vi "Main.vi"(11 "Module Admin":refnum<class "Delacor_lib_QMH_Module Admin.lvclass">) -> ()   [LabVIEW 2024, in "Singleton Subpanel.lvlib"]
doc: "This template is based off of the Queued Message Handler design pattern and the Queued Message Handler project template that ships with LabVIEW.\n\nThe main difference is that the queue is private to this module and communication between modules is performed via Broadcast and Request events.\n\nRequest events are wrapped in public API methods and are handled in the Event Handling Loop (EHL) of this VI. Any module can register for Broadcast events sent by this module. The EHL generates messages based on user interface actions.\n\nThe Message Handling Loop (MHL) processes messages generated by the EHL, or by other messages. The messages are string values, so new messages can be added easily to the Message Cases case structure in the MHL. Each message cluster can also provide an optional value for Message Data, which is a variant that can be converted to whatever message-specific data is required.\n_____\nBased on DQMH Dev Tools: Project Template 7.1.0.1499."
uses:
  Singleton Subpanel.lvlib
  <vilib>/Delacor/Delacor QMH/Libraries/Module Admin_class/Delacor_lib_QMH_Module Admin.lvclass
  Module Data--cluster.ctl
  <vilib>/Delacor/Delacor QMH/Libraries/Message Queue_class/Delacor_lib_QMH_Message Queue.lvclass/Delacor_lib_QMH_Message Queue.ctl
  Stop Argument--cluster.ctl
  <vilib>/Delacor/Delacor QMH/Libraries/Module Admin_class/Delacor_lib_QMH_Module Admin.lvclass/Delacor_lib_QMH_Module Admin.ctl
  Draw FP in SubPanel Argument--cluster.ctl
  Remove from SubPanel Argument--cluster.ctl
  <vilib>/Utility/miscctls.llb/LVPointTypeDef.ctl
  <vilib>/Delacor/Delacor QMH/Libraries/Message Queue_class/Delacor_lib_QMH_Enqueue Message (Single).vi
  <vilib>/Delacor/Delacor QMH/Libraries/Module Admin_class/Delacor_lib_QMH_Get External Launch.vi
  <vilib>/Delacor/Delacor QMH/Libraries/Message Queue_class/Delacor_lib_QMH_Message Queue.lvclass
panel:
  out "error out":errorcluster
  out "Status":string
  in  "Simulate MHL Error":bool
  in  "Simulate EHL Error":bool
  # "Other processes communicate with this Module via its Public API (wrappers for its Request Events).\n\nThis Module communicates with other processes via its Broadcast Events.\nAny process that wants to receive these messages can register for this module's Broadcast events."
  # "This template is for the DQMH framework. See the block diagram for more information on how to use this template."
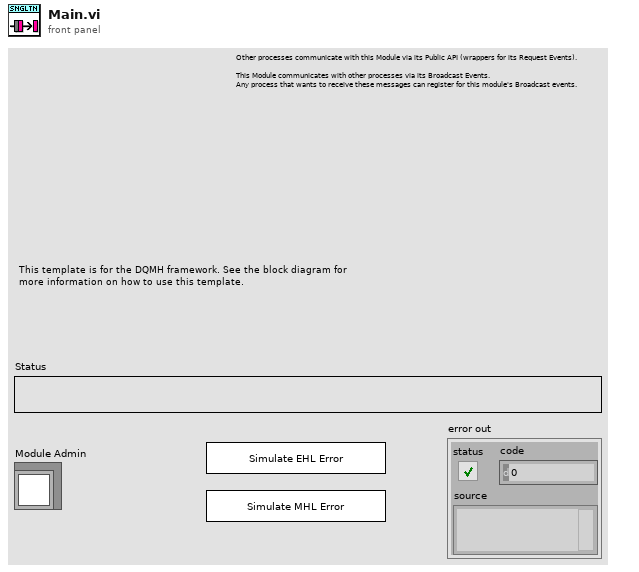
[diagram p1: front panel]
types:
  T1 = typedef "Singleton Subpanel.lvlib/Request Events--cluster.ctl" = cluster{"Stop Module":refnum<user-event>, "Show Panel":refnum<user-event>, "Hide Panel":refnum<user-event>, "Get Module Execution Status":refnum<user-event>, "Show Diagram":refnum<user-event>, "Draw FP in SubPanel":refnum<user-event>, "Remove from SubPanel":refnum<user-event>}
  T2 = typedef "Singleton Subpanel.lvlib/Module Data--cluster.ctl" = cluster{"Status":string, "Sub Panel":refnum<vi>}
  T3 = enum32{"invalid lock state", "Not Locked", "Locked (No Password)", "Password-protected"}
  T4 = typedef "Singleton Subpanel.lvlib/Stop Argument--cluster.ctl" = cluster{"Origin":string, "Exit via Stop Module Req?":bool, "Wait for Module to stop?":bool}
  T5 = typedef "Singleton Subpanel.lvlib/Draw FP in SubPanel Argument--cluster.ctl" = cluster{"Sub Panel":refnum<vi>}
  T6 = typedef "Singleton Subpanel.lvlib/Remove from SubPanel Argument--cluster.ctl" = cluster{"Boolean":bool}
  T7 = typedef "LVPointTypeDef.ctl" = cluster{"Horizontal":i16, "Vertical":i16}
  T8 = enum32{"Invalid", "Standard", "Closed", "Hidden", "Minimized", "Maximized"}
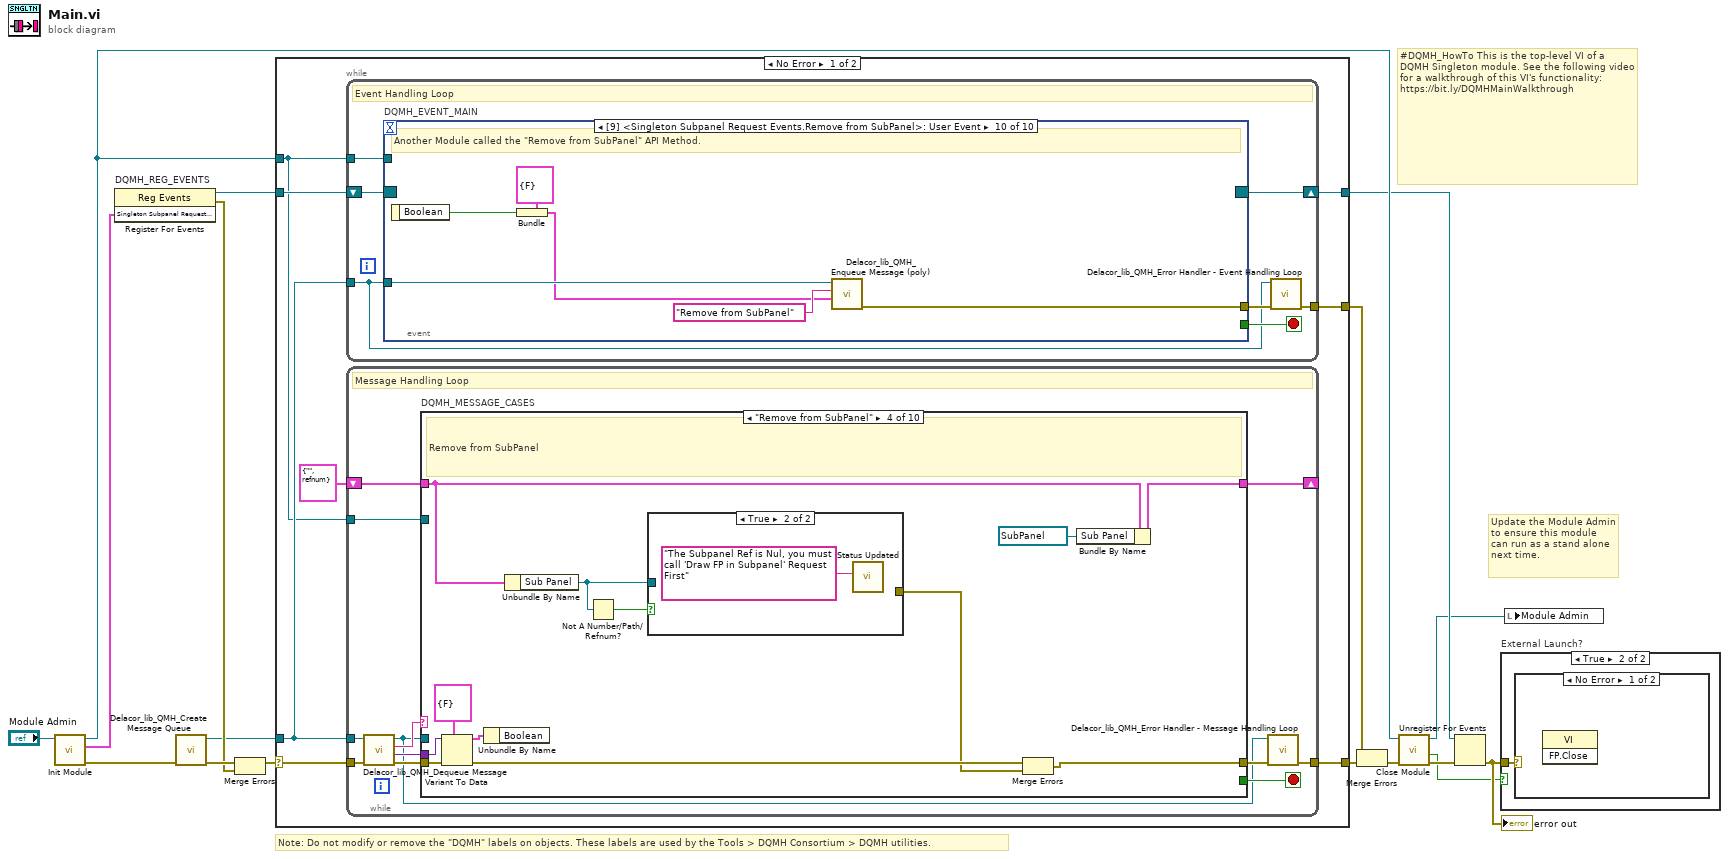
[diagram p0: block diagram]
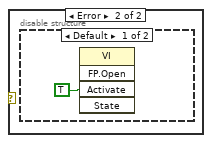
[diagram p3: hidden frame]
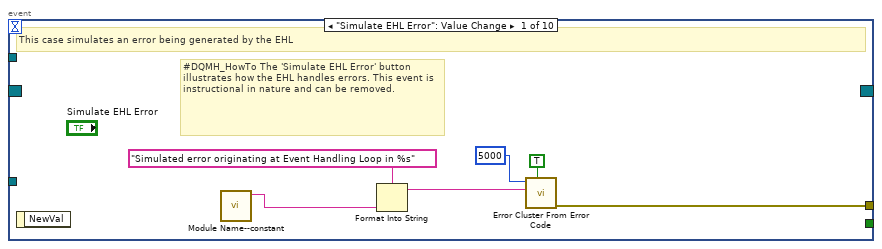
[diagram p5: hidden frame]
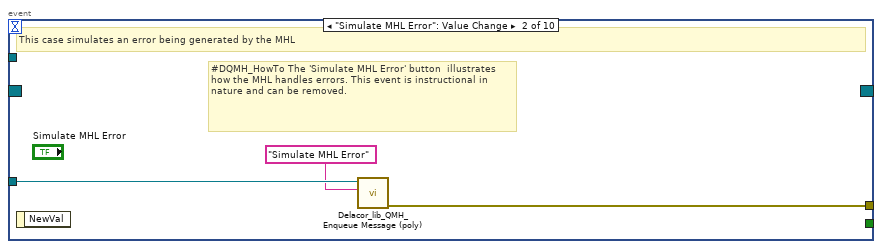
[diagram p6: hidden frame]
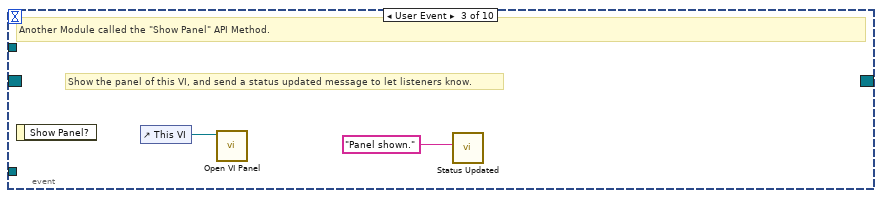
[diagram p7: hidden frame]
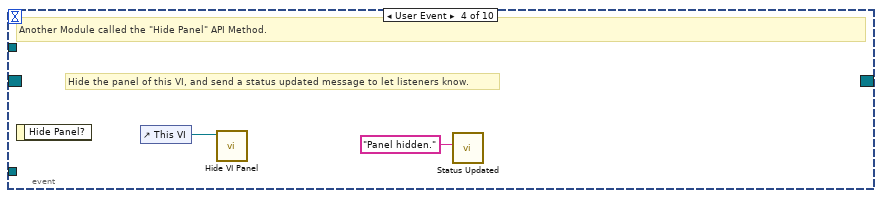
[diagram p8: hidden frame]
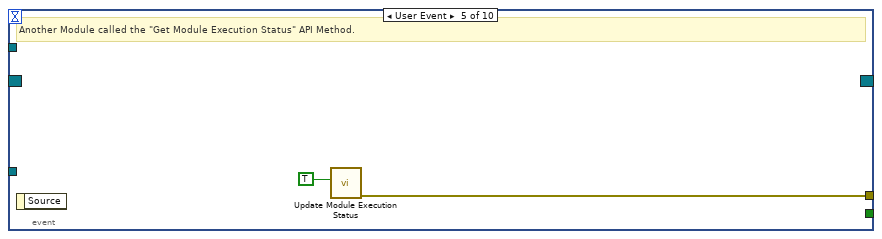
[diagram p9: hidden frame]
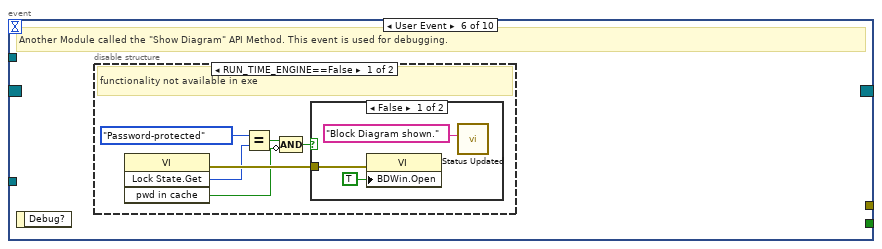
[diagram p10: hidden frame]
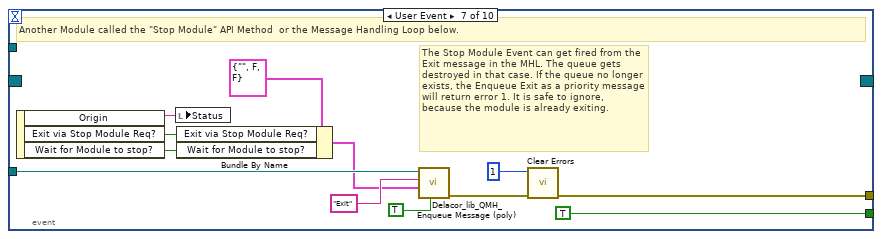
[diagram p13: hidden frame]
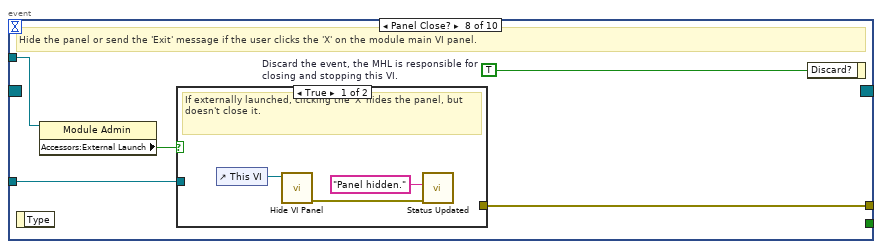
[diagram p14: hidden frame]
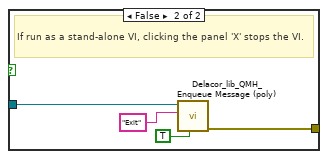
[diagram p15: hidden frame]
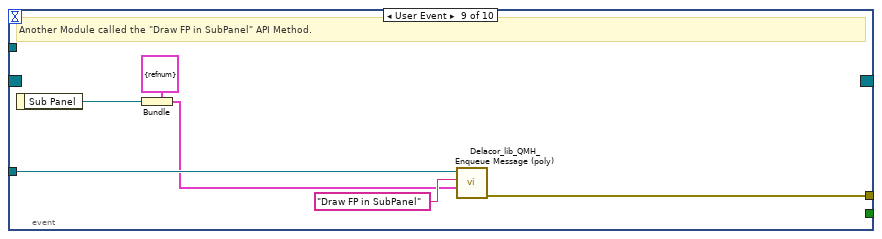
[diagram p16: hidden frame]
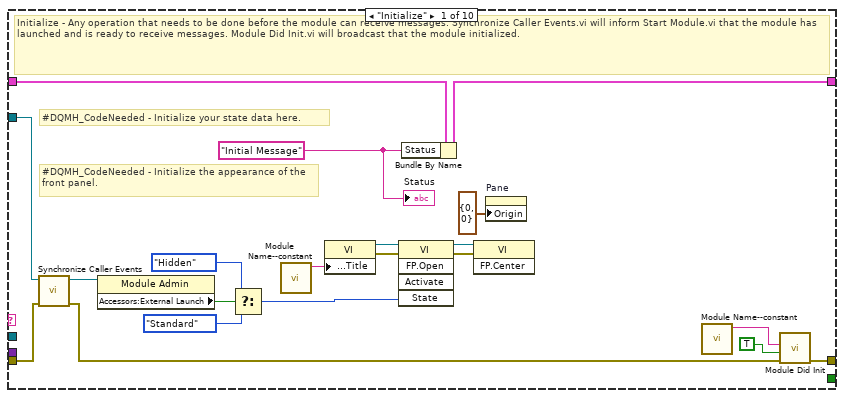
[diagram p17: hidden frame]
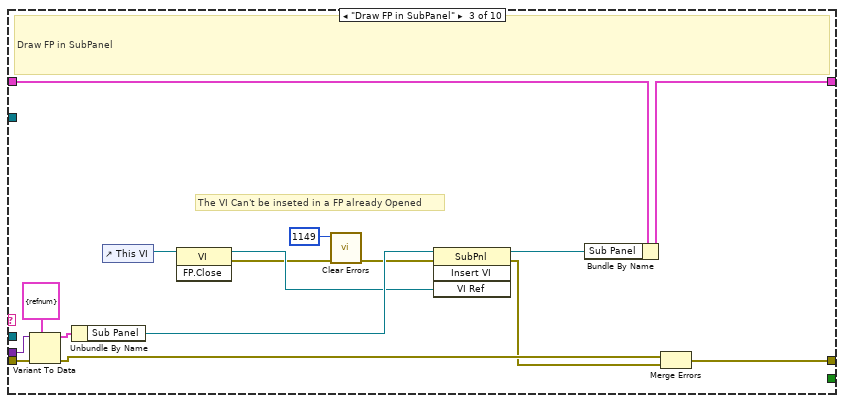
[diagram p19: hidden frame]
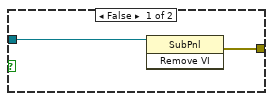
[diagram p20: hidden frame]
diagram:
  # "#DQMH_HowTo This is the top-level VI of a DQMH Singleton module. See the following video for a walkthrough of this VI's functionality: https://bit.ly/DQMHMainWalkthrough"
  # "Note: Do not modify or remove the \"DQMH\" labels on objects. These labels are used by the Tools > DQMH Consortium > DQMH utilities."
  # "Update the Module Admin to ensure this module can run as a stand alone next time."
  n1 = call "Init Module.vi"("Singleton Module Admin in"="Module Admin") -> ("error out"=w16:errorcluster, "Singleton Subpanel Request Events"=w5:T1, "Singleton Module Admin out"=w8:refnum<class "Delacor_lib_QMH_Module Admin.lvclass">)  [unwired: 8 in]
  n2 = register-events "DQMH_REG_EVENTS"(w5) -> (reference out=w6:refnum<event-registration>, error out=w9:errorcluster)  [unwired: 2 in]
  n3 = call <vilib>:"Delacor_lib_QMH_Create Message Queue.vi"("error in"=w16) -> ("error out"=w11:errorcluster, "Message Queue"=w4:refnum<class "Delacor_lib_QMH_Message Queue.lvclass">)  [unwired: 9 in]
  n4 = Merge Errors(w11, w9) -> (w10:errorcluster)
  n5 = case shown="No Error" w10 {
    selector: w10 -> [w23 w222]
    tunnel: [w25 w221] -> w17
    tunnel: [w22 w220] -> w7
    tunnel: w6 -> [w20 w220]
    tunnel: w4 -> [w19 w215]
    tunnel: [w24 _] -> w14
    tunnel: w8 -> [w18 w216]
    frame No Error {
      n6 = while {
        tunnel: w19 -> [w26]
        shift-right: [w29] -> w22
        shift-left: w20 -> [w30]
        tunnel: [w31] -> w24
        tunnel: w18 -> [w27]
        stop <- w28 stop-if-true
        # "Event Handling Loop"
        n7 = event "DQMH_EVENT_MAIN" shown="[9] <Singleton Subpanel Request Events.Remove from SubPanel>: User Event" {
          selector: w30 -> [_ _ _ _ _ _ _ _ _ _]
          dyn-events: [_ _ _ _ _ _ _ _ _ _] -> w29
          timeout: _ -> [_ _ _ _ _ _ _ _ _ _]
          tunnel: [_ _ _ _ _ _ TRUE ("Discard?") _ _ _] -> w28
          tunnel: w26 -> [_ w40 _ _ _ _ w64 w71 w86 w92]
          tunnel: [w38 w41 _ _ w47 _ w67 w73 w81 w87] -> w32
          tunnel: w27 -> [_ _ _ _ _ _ _ w70 _ _]
          event "Simulate EHL Error": Value Change {
            # "#DQMH_HowTo The 'Simulate EHL Error' button  illustrates how the EHL handles errors. This event is instructional in nature and can be removed."
            # "This case simulates an error being generated by the EHL"
            n8 = event-data() -> ()  [unwired: 1 in, 1 out]
            n9 = call "Module Name--constant.vi"() -> ("Module Name"=w35:string)  [unwired: 11 in]
            n10 = Format Into String(format string="Simulated error originating at Event Handling Loop in %s", w35) -> (resulting string=w36:string)  [unwired: 2 in, 1 out]
            n11 = call <vilib>:"Error Cluster From Error Code.vi"("show call chain? (False)"=TRUE, "error message (\"\")"=w36, "error code (0)"=5000) -> ("error out"=w38:errorcluster)  [unwired: 6 in]
          }
          event "Simulate MHL Error": Value Change {
            # "#DQMH_HowTo The 'Simulate MHL Error' button  illustrates how the MHL handles errors. This event is instructional in nature and can be removed."
            # "This case simulates an error being generated by the MHL"
            n12 = event-data() -> ()  [unwired: 1 in, 1 out]
            n13 = call-poly <vilib>:"Delacor_lib_QMH_Enqueue Message (poly).vi"("Message"="Simulate MHL Error", "Message Queue in"=w40) -> ("error out"=w41:errorcluster)  [unwired: 8 in, 1 out]
          }
          event User Event {
            # "Show the panel of this VI, and send a status updated message to let listeners know."
            # "Another Module called the \"Show Panel\" API Method."
            n14 = event-data() -> ()  [unwired: 1 in, 1 out]
            n15 = control-ref of="This VI"() -> (w43:refnum<vi>)
            n16 = call "Open VI Panel.vi"("VI"=w43) -> ()  [unwired: 10 in, 1 out]
            n17 = call "Status Updated.vi"("Status"="Panel shown." ("format string")) -> ()  [unwired: 10 in, 1 out]
          }
          event User Event {
            # "Hide the panel of this VI, and send a status updated message to let listeners know."
            # "Another Module called the \"Hide Panel\" API Method."
            n18 = event-data() -> ()  [unwired: 1 in, 1 out]
            n19 = control-ref of="This VI"() -> (w45:refnum<vi>)
            n20 = call "Hide VI Panel.vi"("VI"=w45) -> ()  [unwired: 10 in, 1 out]
            n21 = call "Status Updated.vi"("Status"="Panel hidden." ("format string")) -> ()  [unwired: 10 in, 1 out]
          }
          event User Event {
            # "Another Module called the \"Get Module Execution Status\" API Method."
            n22 = event-data() -> ()  [unwired: 1 in, 1 out]
            n23 = call "Update Module Execution Status.vi"("Running?"=TRUE) -> ("error out"=w47:errorcluster)  [unwired: 10 in]
          }
          event User Event {
            # "Another Module called the \"Show Diagram\" API Method. This event is used for debugging."
            n24 = event-data() -> ()  [unwired: 1 in, 1 out]
            n25 = disable-structure shown="RUN_TIME_ENGINE==False" {
              frame condition #0 (active) {
                # "functionality not available in exe"
                n26 = invoke on="Invoke Node" class="VI" method="Lock State.Get"() -> (error out=w53:errorcluster, "Get Lock State"=w52:T3, "pwd in cache"=w49:bool)  [unwired: 4 in, 1 out]
                n27 = Equal?(x=T3."Password-protected", y=w52) -> (x = y?=w50:bool)
                n28 = Compound Arithmetic op=AND(w50, invert w49) -> (w48:bool)
                n29 = case shown="False" w48 {
                  tunnel: w53 -> [w56 _]
                  frame False {
                    n30 = property on="Property Node" class="VI"(error in=w56, "BDWin.Open"=TRUE ("Block Diagram Window:Open")) -> ()  [unwired: 1 in, 2 out]
                    n31 = call "Status Updated.vi"("Status"="Block Diagram shown." ("format string")) -> ()  [unwired: 10 in, 1 out]
                  }
                  frame True {
                    # "Password-protected VI, and the password is not in the cache. Do not show the diagram."
                  }
                }
              }
              frame condition #1 {
              }
            }
          }
          event User Event {
            # "The Stop Module Event can get fired from the Exit message in the MHL. The queue gets destroyed in that case. If the queue no longer exists, the Enqueue Exit as a priority message will return error 1. It is safe to ignore, because the module is already exiting."
            # "Another Module called the \"Stop Module\" API Method  or the Message Handling Loop below."
            n32 = event-data() -> ("Origin"=w63:string, "Exit via Stop Module Req?"=w59:bool, "Wait for Module to stop?"=w58:bool)  [unwired: 1 in]
            n33 = local write "Status"(w63) -> ()
            n34 = Bundle By Name(cluster=T4 {"Origin"="", "Exit via Stop Module Req?"=FALSE, "Wait for Module to stop?"=FALSE} ("Stop Argument"), "Exit via Stop Module Req?"=w59, "Wait for Module to stop?"=w58) -> (w57:T4)
            n35 = call-poly <vilib>:"Delacor_lib_QMH_Enqueue Message (poly).vi"("Priority Message? (F)"=TRUE, "Message Data"=w57, "Message"="Exit", "Message Queue in"=w64) -> ("error out"=w68:errorcluster)  [unwired: 6 in, 1 out]
            n36 = call <vilib>:"Clear Errors.vi"("error in (no error)"=w68, "specific error code to clear (0: all)"=1) -> ("error out"=w67:errorcluster)  [unwired: 4 in, 1 out]
          }
          event Panel Close? {
            w72 = TRUE  # Discard the event, the MHL is responsible for closing and stopping this VI.
            # "Hide the panel or send the 'Exit' message if the user clicks the 'X' on the module main VI panel."
            n37 = event-data() -> ()  [unwired: 1 in, 1 out]
            n38 = property on="Property Node" class="Module Admin"(reference=w70) -> ("Accessors:External Launch"=w69:bool)  [unwired: 1 in, 2 out]
            n39 = case shown="True" w69 {
              tunnel: w71 -> [_ w79]
              tunnel: [_ w80] -> w73
              frame True {
                # "If externally launched, clicking the 'X' hides the panel, but doesn't close it."
                n40 = control-ref of="This VI"() -> (w76:refnum<vi>)
                n41 = call "Hide VI Panel.vi"("VI"=w76) -> ("error out"=w74:errorcluster)  [unwired: 10 in]
                n42 = call "Status Updated.vi"("error in"=w74, "Status"="Panel hidden." ("format string")) -> ()  [unwired: 9 in, 1 out]
              }
              frame False {
                # "If run as a stand-alone VI, clicking the panel 'X' stops the VI."
                n43 = call-poly <vilib>:"Delacor_lib_QMH_Enqueue Message (poly).vi"("Priority Message? (F)"=TRUE, "Message"="Exit", "Message Queue in"=w79) -> ("error out"=w80:errorcluster)  [unwired: 7 in, 1 out]
              }
            }
            n44 = event-data ("Event Filter Node")("Discard?"=w72) -> ()  [unwired: 1 in, 1 out]
          }
          event User Event {
            # "Another Module called the \"Draw FP in SubPanel\" API Method."
            n45 = event-data() -> ("Sub Panel"=w82:refnum<vi>)  [unwired: 1 in]
            n46 = Bundle(cluster=T5 {"Sub Panel"=refnum} ("Draw FP in SubPanel Argument"), "Sub Panel"=w82) -> (w83:T5)
            n47 = call-poly <vilib>:"Delacor_lib_QMH_Enqueue Message (poly).vi"("Message Data"=w83, "Message"="Draw FP in SubPanel", "Message Queue in"=w86) -> ("error out"=w81:errorcluster)  [unwired: 7 in, 1 out]
          }
          event User Event {
            # "Another Module called the \"Remove from SubPanel\" API Method."
            n48 = event-data() -> ("Boolean"=w88:bool)  [unwired: 1 in]
            n49 = Bundle(cluster=T6 {"Boolean"=FALSE} ("Remove from SubPanel Argument"), "Boolean"=w88) -> (w89:T6)
            n50 = call-poly <vilib>:"Delacor_lib_QMH_Enqueue Message (poly).vi"("Message Data"=w89, "Message"="Remove from SubPanel", "Message Queue in"=w92) -> ("error out"=w87:errorcluster)  [unwired: 7 in, 1 out]
          }
        }
        n51 = call-dynamic "Delacor_lib_QMH_Error Handler - Event Handling Loop.vi"("error in"=w32, "Message Queue in"=w26) -> ("dup error in"=w31:errorcluster)  [unwired: 8 in, 1 out]
      }
      n52 = while {
        tunnel: w19 -> [w93]
        shift-right: [w101] -> _
        shift-left: T2 {"Status"="", "Sub Panel"=refnum} ("Data Cluster") -> [w102]
        tunnel: w23 -> [w104]
        tunnel: [w96] -> w25
        tunnel: w18 -> [w97]
        stop <- w100 stop-if-true
        # "Message Handling Loop"
        n53 = call-dynamic "Delacor_lib_QMH_Dequeue Message.vi"("error in"=w104, "Message Queue in"=w93) -> ("error out"=w103:errorcluster, "Message Data"=w98:variant, "Message"=w99:string, "Message Queue out"=w94:refnum<class "Delacor_lib_QMH_Message Queue.lvclass">)  [unwired: 6 in]
        n54 = case "DQMH_MESSAGE_CASES" shown="\"Remove from SubPanel\"" w99 {
          selector: w99 -> [_ _ _ _ _ _ _ _ _ w210]
          tunnel: w94 -> [_ _ _ _ _ _ _ w175 w198 _]
          tunnel: w103 -> [w122 w126 w142 w154 w160 w162 w171 w182 w204 w213]
          tunnel: [w120 w126 w132 w148 w159 w162 w170 w178 w199 w214] -> w95
          tunnel: w102 -> [w111 w125 w141 w149 w158 w161 w168 w177 w190 w211]
          tunnel: [w110 w125 w128 w144 w158 w161 w168 w177 w190 w211] -> w101
          tunnel: [_ _ _ _ _ _ _ _ w197 _] -> w100
          tunnel: w98 -> [_ _ w140 w152 _ _ _ w176 w196 _]
          tunnel: w97 -> [w112 _ _ _ _ _ _ w174 w191 _]
          frame "Initialize" {
            w106 = "Initial Message" ("Initial Message")
            # "#DQMH_CodeNeeded - Initialize the appearance of the front panel."
            # "#DQMH_CodeNeeded - Initialize your state data here."
            # "Initialize - Any operation that needs to be done before the module can receive messages. Synchronize Caller Events.vi will inform Start Module.vi that the module has launched and is ready to receive messages. Module Did Init.vi will broadcast that the module initialized."
            n55 = call "Synchronize Caller Events.vi"("error in"=w122, "Singleton Module Admin in"=w112) -> ("error out"=w121:errorcluster, "Singleton Module Admin out"=w107:refnum<class "Delacor_lib_QMH_Module Admin.lvclass">)  [unwired: 8 in]
            n56 = property on="Property Node" class="Module Admin"(reference=w107) -> ("Accessors:External Launch"=w116:bool)  [unwired: 1 in, 2 out]
            n57 = Select(t=T8."Hidden" ("State"), s=w116, f=T8."Standard" ("State")) -> (s? t:f=w113:T8)
            n58 = call "Module Name--constant.vi"() -> ("Module Name"=w119:string)  [unwired: 11 in]
            n59 = property on="Property Node" class="VI"("Front Panel.Title"=w119) -> (reference out=w118:refnum<vi>, error out=w124:errorcluster)  [unwired: 2 in]
            n60 = invoke on="Invoke Node" class="VI" method="FP.Open"(reference=w118, error in=w124, "State"=w113) -> (reference out=w117:refnum<vi>, error out=w123:errorcluster)  [unwired: 2 in, 3 out]
            n61 = Bundle By Name(cluster=w111, "Status"=w106) -> (w110:T2)
            n62 = invoke on="Invoke Node" class="VI" method="FP.Center"(reference=w117, error in=w123) -> ()  [unwired: 1 in, 3 out]
            n63 = property on="Pane" class="Pane"("Origin"=T7 {"Horizontal"=0, "Vertical"=0}) -> ()  [unwired: 2 in, 2 out]
            n64 = call "Module Name--constant.vi"() -> ("Module Name"=w108:string)  [unwired: 11 in]
            n65 = call "Module Did Init.vi"("error in"=w121, "Initialized?"=TRUE, "Origin"=w108) -> ("error out"=w120:errorcluster)  [unwired: 8 in]
            "Status" <- w106
          }
          frame "---Module Specific---" {
            # "Separator -- The following cases handle messages specific to this Module."
          }
          frame "Draw FP in SubPanel" {
            # "The VI Can't be inseted in a FP already Opened"
            # "Draw FP in SubPanel"
            n66 = Variant To Data(error in=w142, type=T5 {"Sub Panel"=refnum} ("Draw FP in SubPanel Argument"), Variant=w140) -> (data=w138:T5, error out=w131:errorcluster)
            n67 = Unbundle By Name(w138) -> ("Sub Panel"=w136:refnum<vi>)
            n68 = control-ref of="This VI"() -> (w137:refnum<vi>)
            n69 = invoke class="VI" method="FP.Close"(reference=w137) -> (reference out=w135:refnum<vi>, error out=w134:errorcluster)  [unwired: 2 in, 1 out]
            n70 = call <vilib>:"Clear Errors.vi"("error in (no error)"=w134, "specific error code to clear (0: all)"=1149) -> ("error out"=w133:errorcluster)  [unwired: 4 in, 1 out]
            n71 = invoke class="SubPnl" method="Insert VI"(reference=w136, error in=w133, "VI Ref"=w135) -> (reference out=w127:refnum<vi>, error out=w130:errorcluster)  [unwired: 1 in, 2 out]
            n72 = Bundle By Name(cluster=w141, "Sub Panel"=w127) -> (w128:T2)
            n73 = Merge Errors(w131, w130) -> (w132:errorcluster)
          }
          frame "Remove from SubPanel" {
            # "Remove from SubPanel"
            n74 = Variant To Data(error in=w154, type=T6 {"Boolean"=FALSE} ("Remove from SubPanel Argument"), Variant=w152) -> (data=w150:T6, error out=w153:errorcluster)
            n75 = Unbundle By Name(w150) -> ()  [unwired: 1 out]
            n76 = Unbundle By Name(w149) -> ("Sub Panel"=w146:refnum<vi>)
            n77 = Not A Number/Path/Refnum?(number/path/refnum=w146) -> (NaN/Path/Refnum?=w145:bool)
            n78 = case shown="True" w145 {
              tunnel: w146 -> [w156 _]
              tunnel: [w155 _] -> w147
              frame False {
                n79 = invoke class="SubPnl" method="Remove VI"(reference=w156) -> (error out=w155:errorcluster)  [unwired: 2 in, 2 out]
              }
              frame True {
                n80 = call "Status Updated.vi"("Status"="The Subpanel Ref is Nul, you must call 'Draw FP in Subpanel' Request First") -> ()  [unwired: 10 in, 1 out]
              }
            }
            n81 = Merge Errors(w153, w147) -> (w148:errorcluster)
            n82 = Bundle By Name(cluster=w149, "Sub Panel"=refnum<vi> refnum) -> (w144:T2)
          }
          frame "---Copy This Frame---" {
            # "Duplicate this frame when creating new messages.  Change this comment in the duplicated frame to describe this message."
            n83 = Merge Errors(w160) -> (w159:errorcluster)
          }
          frame "---Exit and Error Handling---" {
            # "Separator - The following cases handle errors and exit messages."
          }
          frame "Simulate MHL Error" {
            # "#DQMH_HowTo The 'Simulate MHL Error' button  illustrates how the MHL handles errors. This event is instructional in nature and can be removed."
            # "Simulate an error occurring at the MHL"
            n84 = call "Module Name--constant.vi"() -> ("Module Name"=w164:string)  [unwired: 11 in]
            n85 = Format Into String(format string="Simulated error originating at Message Handling Loop in %s", w164) -> (resulting string=w165:string)  [unwired: 2 in, 1 out]
            n86 = call <vilib>:"Error Cluster From Error Code.vi"("show call chain? (False)"=TRUE, "error message (\"\")"=w165, "error code (0)"=5001) -> ("error out"=w169:errorcluster)  [unwired: 6 in]
            n87 = Merge Errors(w171, w169) -> (w170:errorcluster)
          }
          frame "Error" {
            # "#DQMH_CodeRecommended - If the module is running in standalone mode (External Launch = FALSE), this code will pop up an error dialog and call the 'Exit' message if an error occurs. Add more fine-grained error management here."
            # "Error - Check the error message data and respond accordingly. This message is sent by the \"Error Handler\" VIs at the end of each loop in this application."
            n88 = property on="Property Node" class="Module Admin"(reference=w174) -> ("Accessors:External Launch"=w173:bool)  [unwired: 1 in, 2 out]
            n89 = Variant To Data(error in=w182, type=errorcluster {"status"=FALSE, "code"=0, "source"=""} ("error constant"), Variant=w176) -> (data=w172:errorcluster, error out=w180:errorcluster)
            n90 = local write "error out"(w172) -> ()
            n91 = call "Error Reported.vi"("Error"=w172) -> ()  [unwired: 10 in, 1 out]
            n92 = case shown="False" w173 {
              tunnel: [w187 _] -> w179
              tunnel: w175 -> [w185 _]
              tunnel: w172 -> [w186 _]
              frame False {
                n93 = disable-structure shown="Default" {
                  disable-tunnel: w186 -> [w188 _]
                  frame condition #0 (active) {
                    # "If the module is running standalone, then pop up an error dialog and call the \"Exit\" message."
                    n94 = call <vilib>:"Simple Error Handler.vi"("error in (no error)"=w188) -> ()  [unwired: 4 in, 5 out]
                  }
                  frame condition #1 {
                    # "To prevent the Simple Error Handler VI from being loaded (e.g. when deploying to a Real-Time target), add the Conditional Disable Symbol \"DQMH_Disable_SEH\" to your project and set it to TRUE."
                  }
                }
                n95 = call-poly <vilib>:"Delacor_lib_QMH_Enqueue Message (poly).vi"("Priority Message? (F)"=TRUE, "Message"="Exit", "Message Queue in"=w185) -> ("error out"=w187:errorcluster)  [unwired: 7 in, 1 out]
              }
              frame True {
                # "If the module was launched externally, calling the Error Reported broadcast VI is the only action performed by the \"Error\" message. The module's caller can then process the error appropriately."
              }
            }
            n96 = Merge Errors(w180, w179) -> (w178:errorcluster)
          }
          frame "Exit" {
            w195 = 91  # 91: not all Exit messages will have an argument
            w197 = TRUE  # Stop the VI
            # "Release the message queue reference"
            # "#DQMH_CodeNeeded - Add any required cleanup code here."
            # "Exit - Exit the application."
            n97 = Variant To Data(error in=w204, type=T4 {"Origin"="", "Exit via Stop Module Req?"=FALSE, "Wait for Module to stop?"=FALSE} ("Stop Argument"), Variant=w196) -> (data=w193:T4, error out=w201:errorcluster)
            n98 = call <vilib>:"Clear Errors.vi"("error in (no error)"=w201, "specific error code to clear (0: all)"=w195) -> ("error out"=w203:errorcluster)  [unwired: 4 in, 1 out]
            n99 = control-ref of="This VI"() -> (w192:refnum<vi>)
            n100 = call-dynamic "Delacor_lib_QMH_Release Message Queue.vi"("error in"=w203, "Message Queue"=w198) -> ("error out"=w202:errorcluster)  [unwired: 9 in]
            n101 = call "Handle Exit.vi"("Stop Argument"=w193, "Admin in"=w191, "VI reference"=w192) -> ("error out"=w200:errorcluster)  [unwired: 7 in, 1 out]
            n102 = Merge Errors(w202, w200) -> (w199:errorcluster)
            n103 = Unbundle By Name(w190) -> ("Sub Panel"=w189:refnum<vi>)
            n104 = call "Error Reported.vi"("Error"=w199) -> ()  [unwired: 10 in, 1 out]
            n105 = invoke class="SubPnl" method="Remove VI"(reference=w189) -> ()  [unwired: 2 in, 3 out]
          }
          frame Default {
            # "'Default' case only runs if there is a message that isn't defined in any of the other cases.  Output a programming error."
            n106 = call "Module Name--constant.vi"() -> ("Module Name"=w209:string)  [unwired: 11 in]
            n107 = Format Into String(format string="The invalid message string \"%s\" was received in the Message Handling Loop for module \"%s\".", w210, w209) -> (resulting string=w205:string)  [unwired: 2 in, 1 out]
            n108 = call <vilib>:"Error Cluster From Error Code.vi"("show call chain? (False)"=TRUE, "error message (\"\")"=w205, "error code (0)"=1) -> ("error out"=w212:errorcluster)  [unwired: 6 in]
            n109 = Merge Errors(w213, w212) -> (w214:errorcluster)
          }
        }
        n110 = call-dynamic "Delacor_lib_QMH_Error Handler - Message Handling Loop.vi"("error in"=w95, "Message Queue in"=w94) -> ("dup error in"=w96:errorcluster)  [unwired: 8 in, 1 out]
      }
    }
    frame Error {
      # "Synchronize Caller Events.vi will inform Start Module.vi that the module has launched and will let the code calling Start Module.vi register for broadcasts and would permit the caller receive the broadcast that an error occurred at launch time."
      n111 = call-dynamic "Delacor_lib_QMH_Release Message Queue.vi"("error in"=w222, "Message Queue"=w215) -> ("error out"=w221:errorcluster)  [unwired: 9 in]
      n112 = call "Synchronize Caller Events.vi"("Singleton Module Admin in"=w216) -> ("error out"=w223:errorcluster)  [unwired: 9 in, 1 out]
      n113 = call "Module Name--constant.vi"() -> ("Module Name"=w219:string)  [unwired: 11 in]
      n114 = Format Into String(format string="An error occurred during initialization. %s is no longer running.", w219) -> (resulting string=w217:string)  [unwired: 2 in, 1 out]
      n115 = Merge Errors(w221, w223) -> (w224:errorcluster)
      n116 = call "Error Reported.vi"("Additional Information"=w217, "Error"=w224) -> ()  [unwired: 9 in, 1 out]
    }
  }
  n117 = Merge Errors(w14, w17) -> (w13:errorcluster)
  n118 = call "Close Module.vi"("error in"=w13, "Module Admin in"=w8) -> ("error out"=w15:errorcluster, "External Launch"=w1:bool, "Module Admin out"=w2:refnum<class "Delacor_lib_QMH_Module Admin.lvclass">)  [unwired: 7 in]
  n119 = Unregister For Events(event registration refnum=w7, error in=w15) -> (error out=w12:errorcluster)
  "error out" <- w12
  n120 = case "External Launch?" shown="True" w1 {
    tunnel: w12 -> [_ w225]
    frame False {
    }
    frame True {
      n121 = case shown="No Error" w225 {
        frame No Error {
          n122 = invoke on="Invoke Node" class="VI" method="FP.Close"() -> ()  [unwired: 3 in, 3 out]
        }
        frame Error {
          n123 = disable-structure shown="Default" {
            frame condition #0 (active) {
              n124 = invoke class="VI" method="FP.Open"("Activate"=TRUE ("Activate?")) -> ()  [unwired: 4 in, 5 out]
            }
            frame condition #1 {
              # "Don't show panel on error if running inside a built EXE."
            }
          }
        }
      }
    }
  }
  n125 = local write "Module Admin"(w2) -> ()
